vi "DSF.Engine.Sequencer.Get Active Plugin Indicies.vi"(8 "error in (no error)":errorcluster, 10 "engine iteration":u64, 11 "Sequencer in":refnum<class "DSF.Engine.Sequencer.lvclass">) -> (0 "error out":errorcluster, 2 "active Plugin indicies":i32[](array[numeric]), 3 "Sequencer out":refnum<class "DSF.Engine.Sequencer.lvclass">)   [LabVIEW 2016, in "DSF.Engine.lvlib" / "DSF.Engine.Sequencer.lvclass"]
uses:
  DSF.Engine.Sequencer.lvclass
  DSF.Engine.Sequencer.lvclass/DSF.Engine.Sequencer.ctl
  Sequencer Bundle.lvclass/Sequencer Bundle.ctl
  Timing/DSF.Engine.Timing.lvclass
  Sequencer Bundle.lvclass
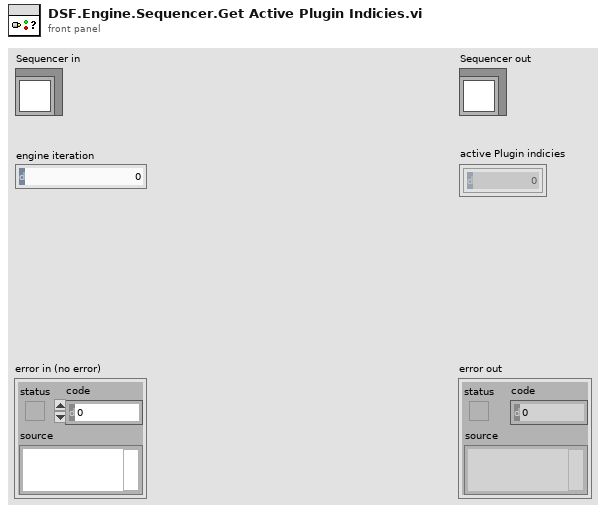
[diagram p1: front panel]
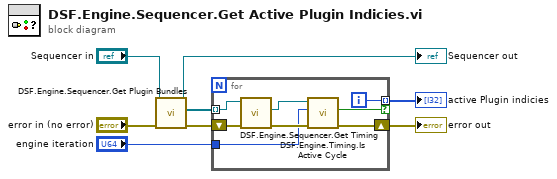
[diagram p0: block diagram]
diagram:
  n1 = call "DSF.Engine.Sequencer.Get Plugin Bundles.vi"("error in (no error)"="error in (no error)", "Sequencer in"="Sequencer in") -> ("error out"=w7:errorcluster, "Plugin Bundles"=w8:refnum<class "Sequencer Bundle.lvclass">[], "Sequencer out"=→"Sequencer out":refnum<class "DSF.Engine.Sequencer.lvclass">)  [unwired: 7 in]
  n2 = for {
    shift-right: [w16] -> w4
    shift-left: w7 -> [w14]
    tunnel: w8 -> [w15] mode=indexing
    tunnel: "engine iteration" -> [w9]
    tunnel: [w11] -> w1 mode=indexing if=w10
    i -> [w11]
    n3 = call "DSF.Engine.Sequencer.Get Timing.vi"("error in (no error)"=w14, "Sequencer Bundle in"=w15) -> ("error out"=w12:errorcluster, "Plugin Timing"=w13:refnum<class "DSF.Engine.Timing.lvclass">)  [unwired: 7 in, 1 out]
    n4 = call "DSF.Engine.Timing.Is Active Cycle.vi"("error in (no error)"=w12, "iteration"=w9, "Execution Timing in"=w13) -> ("error out"=w16:errorcluster, "active?"=w10:bool)  [unwired: 6 in, 1 out]
  }
  "error out" <- w4
  "active Plugin indicies" <- w1
